vi "GenOneOf_Has_Accessor.vi"(7 "application reference":refnum<vi>, 8 "error in (no error)":errorcluster, 10 "message element metadata":T1={"Field Name"="nested_message_2", "Embedded Message Name"="echo_array_NestedMessage2", "Protobuf Index"=3, "MessageElementType"=enum."MessageValue", "Repeated"=FALSE, "Is in Oneof"=TRUE, "Oneof Container Name"="echo_array_NestedMessage_union"}, 11 "path":path) -> (0 "error out":errorcluster)   [LabVIEW 2019, in "gRPC Template Creation Utility.lvlib"]
uses:
  gRPC Template Creation Utility.lvlib
  TypeDefs/Message Element Metadata (Scripting).ctl
  TypeDefs/Message Element Type.ctl
  <vilib>/Utility/traverseref.llb/TRef TravTarget.ctl
  <vilib>/Utility/traverseref.llb/VI Scripting - Traverse.lvlib
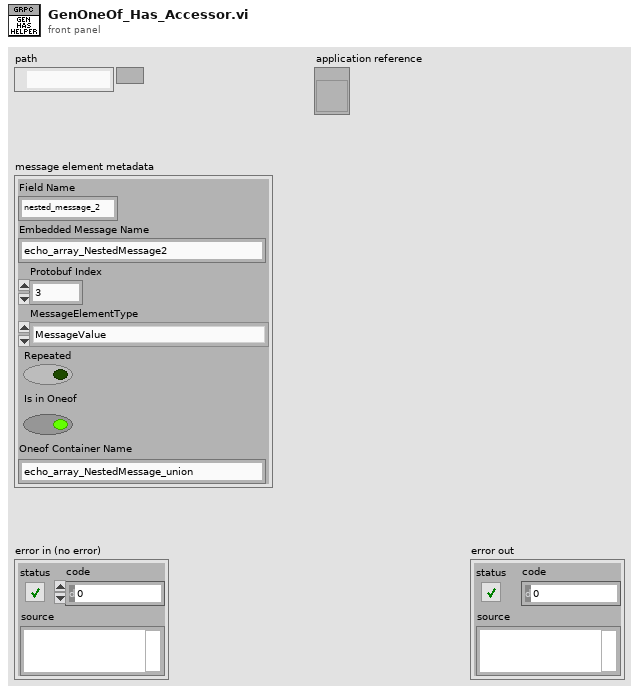
[diagram p1: front panel]
types:
  T1 = typedef "gRPC Template Creation Utility.lvlib/Message Element Metadata (Scripting).ctl" = cluster{"Field Name":string, "Embedded Message Name":string, "Protobuf Index":i32, "MessageElementType":T2, "Repeated":bool, "Is in Oneof":bool, "Oneof Container Name":string}
  T2 = typedef "gRPC Template Creation Utility.lvlib/Message Element Type.ctl" = enum32{"Int32Value", "FloatValue", "DoubleValue", "BoolValue", "StringValue", "MessageValue", "Int64Value", "UInt32Value", "UInt64Value", "EnumValue", "Bytes", "Fixed64", "Fixed32", "SFixed64", "SFixed32", "SInt64", "SInt32"}
  T3 = typedef "TRef TravTarget.ctl" = enum16{"FP", "BD", "Other"}
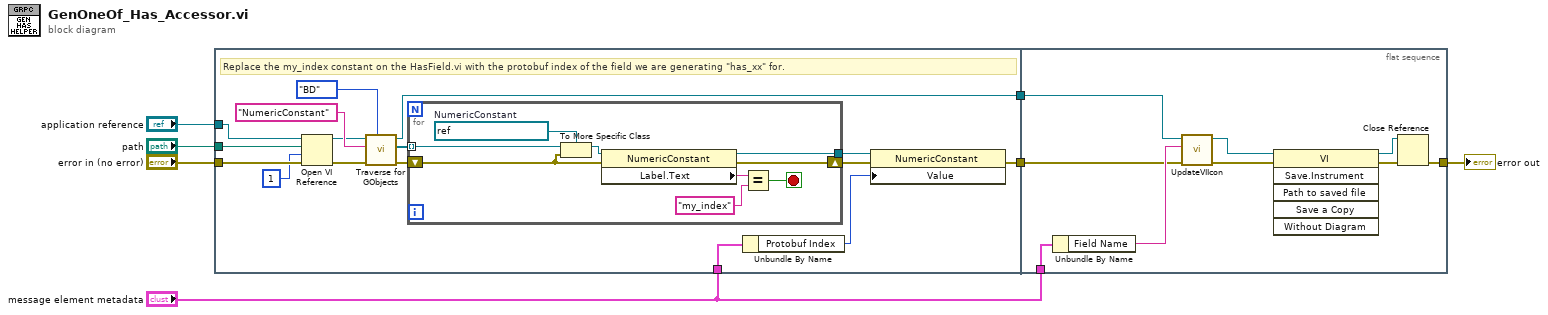
[diagram p0: block diagram]
diagram:
  n1 = flat-sequence {
    tunnel: "error in (no error)" -> [w16]
    tunnel: "path" -> [w15]
    tunnel: [w11] -> w4
    tunnel: [w22] -> w3
    tunnel: "application reference" -> [w10]
    tunnel: "message element metadata" -> [w8]
    tunnel: [w39] -> w7
    tunnel: w4 -> [w34]
    tunnel: w3 -> [w37]
    tunnel: "message element metadata" -> [w35]
    frame #0 {
      # "Replace the my_index constant on the HasField.vi with the protobuf index of the field we are generating \"has_xx\" for."
      n2 = Open VI Reference(application reference (local)=w10, vi path=w15, options=1, error in (no error)=w16) -> (vi reference=w12:refnum<vi>, error out=w19:errorcluster)  [unwired: 2 in]
      n3 = call <vilib>:"Traverse for GObjects.vi"("Traverse Target"=TRef_TravTarget."BD", "error in (no error)"=w19, "Class Name"="NumericConstant", "VI Refnum"=w12) -> ("error out"=w13:errorcluster, "References"=w18:refnum<vi>[], "dup VI Refnum"=w11:refnum<vi>)  [unwired: 4 in, 1 out]
      n4 = for {
        tunnel: w18 -> [w26] mode=indexing
        shift-right: [w28] -> w23
        shift-left: w13 -> [w27]
        tunnel: [w29] -> w17
        stop <- w30 stop-if-true
        w24 = refnum<vi> refnum  # NumericConstant
        n5 = To More Specific Class(target class=w24, reference=w26, error in=w27) -> (specific class reference=w25:refnum<vi>)  [unwired: 1 out]
        n6 = property class="NumericConstant"(reference=w25, error in=w27) -> (reference out=w29:refnum<vi>, error out=w28:errorcluster, "Label.Text"=w32:string)
        n7 = Equal?(x=w32, y="my_index") -> (x = y?=w30:bool)
      }
      n8 = Unbundle By Name(w8) -> ("Protobuf Index"=w9:i32)
      n9 = property class="NumericConstant"(reference=w17, error in=w23, "Value"=w9) -> (error out=w22:errorcluster)  [unwired: 1 out]
    }
    frame #1 {
      n10 = Unbundle By Name(w35) -> ("Field Name"=w38:string)
      n11 = call "UpdateVIIcon.vi"("error in (no error)"=w37, "Method Name"=w38, "VI in"=w34) -> ("error out"=w36:errorcluster, "VI out"=w33:refnum<vi>)  [unwired: 7 in]
      n12 = invoke class="VI" method="Save.Instrument"(reference=w33, error in=w36) -> (reference out=w40:refnum<vi>, error out=w41:errorcluster)  [unwired: 4 in, 4 out]
      n13 = Close Reference(reference=w40, error in (no error)=w41) -> (error out=w39:errorcluster)
    }
  }
  "error out" <- w7
